vi "Memory.Pointer.Internal.New.vi"(8 "error in (no error)":errorcluster, 11 "size":u64 format="%08x bytes") -> (0 "error out":errorcluster, 3 "pointer":refnum<class "Memory.Pointer.Internal.lvclass">)   [LabVIEW 2016, in "Memory.lvlib" / "Memory.Pointer.Internal.lvclass"]
doc: "Allocates a new pointer that points to a block of memory that is <b>size</b> bytes in length."
uses:
  Memory.Pointer.Internal.lvclass
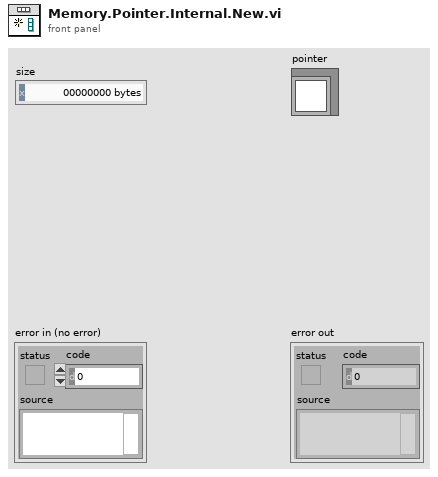
[diagram p1: front panel]
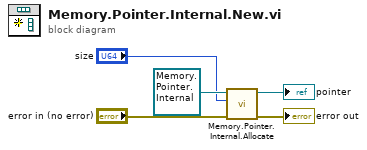
[diagram p0: block diagram]
diagram:
  n1 = call "Memory.Pointer.Internal.Allocate.vi"("error in (no error)"="error in (no error)", "size"="size", "pointer in"=refnum<class "Memory.Pointer.Internal.lvclass"> refnum ("Pointer")) -> ("error out"=→"error out":errorcluster, "pointer out"=→"pointer":refnum<class "Memory.Pointer.Internal.lvclass">)  [unwired: 7 in]
